vi "RefreshTafMenu.vi"(8 "ErrorIn":errorcluster, 11 "ReferenceIn":refnum<class "DemoApplication.lvclass">) -> (0 "ErrorOut":errorcluster, 3 "ReferenceIn":refnum<class "DemoApplication.lvclass">)   [LabVIEW 2021, in "DemoApplication.lvclass"]
uses:
  DemoApplication.lvclass
  .Externals/Library_TAF_ApplicationFramework/MasterGUI/MasterGUI.lvclass
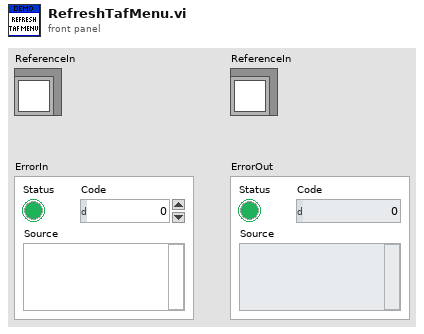
[diagram p1: front panel]
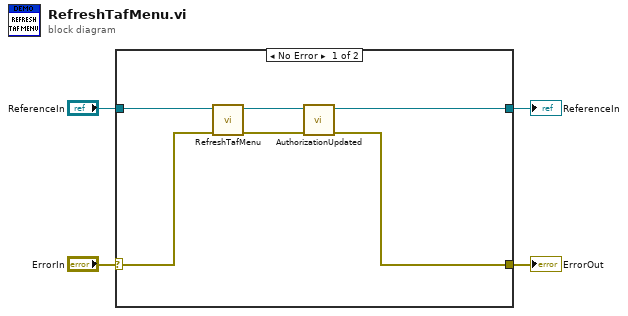
[diagram p0: block diagram]
diagram:
  n1 = case shown="No Error" "ErrorIn" {
    selector: "ErrorIn" -> [w10 w12]
    tunnel: [w8 w12] -> w3
    tunnel: [w5 w11] -> w1
    tunnel: "ReferenceIn" -> [w7 w11]
    frame No Error {
      n2 = call-parent "RefreshTafMenu.vi"("ErrorIn"=w10, "ObjectIn"=w7) -> ("ErrorOut"=w9:errorcluster, "ObjectOut"=w6:refnum<class "DemoApplication.lvclass">)  [unwired: 8 in]
      n3 = call-dynamic "AuthorizationUpdated.vi"("ErrorIn"=w9, "ReferenceIn"=w6) -> ("ErrorOut"=w8:errorcluster, "ReferenceIn"=w5:refnum<class "DemoApplication.lvclass">)  [unwired: 8 in]
    }
    frame Error {
    }
  }
  "ErrorOut" <- w3
  "ReferenceIn" <- w1
